vi "AWS_ConstructQuery.vi"(8 "error in (no error)":errorcluster, 11 "Queries":T1 {"Object Type" items=["File", "Channel Group", "Channel"]; "Operator" items=["=", "<>", ">", "<", ">=", "<=", "#"]}) -> (0 "error out":errorcluster, 3 "Refnum out":T4)   [LabVIEW 2014]
uses:
  <vilib>/userdefined/DFQuery.ctl
  Controls/Query.ctl
  <vilib>/DataFinder/DataTypes/object type.ctl
  <vilib>/DataFinder/DataTypes/comparison operator.ctl
  <vilib>/DataFinder/Create Query (String).vi
  <vilib>/DataFinder/Create Query (Numeric).vi
  <vilib>/DataFinder/NI_DataFinder Toolkit.lvlib
  <vilib>/userdefined/NI_DataFinder Controls.lvlib
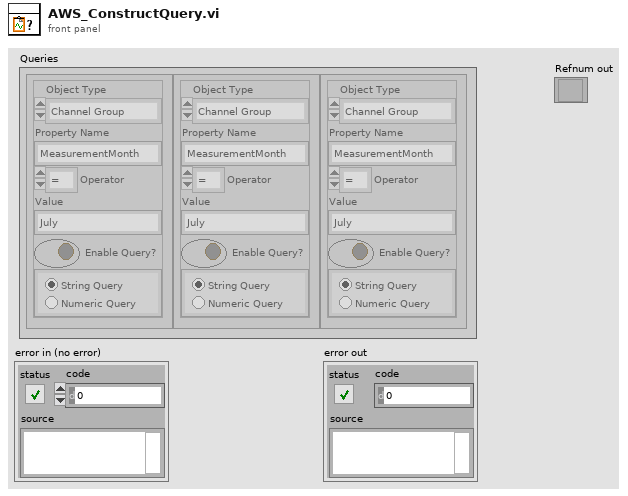
[diagram p1: front panel]
types:
  T1 = typedef "Query.ctl" = cluster{"Object Type":T2, "Property Name":string, "Operator":T3, "Value":string, "Enable Query?":bool, "Radio Buttons":enum32{"Radio Selection 1", "Radio Selection 2"}}[]
  T2 = typedef "NI_DataFinder Toolkit.lvlib/object type.ctl" = u16
  T3 = typedef "NI_DataFinder Toolkit.lvlib/comparison operator.ctl" = u16
  T4 = typedef "NI_DataFinder Controls.lvlib/DFQuery.ctl" = refnum<k20>
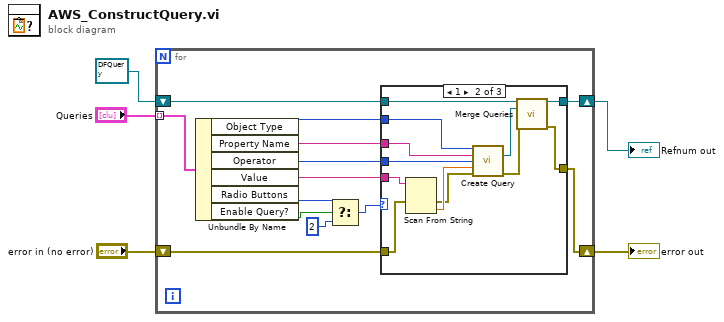
[diagram p0: block diagram]
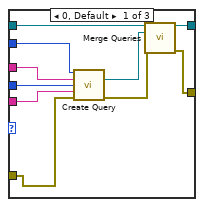
[diagram p2: hidden frame]
diagram:
  n1 = for {
    tunnel: "Queries" -> [w15] mode=indexing
    shift-right: [w17] -> w4
    shift-left: T4 refnum ("query reference out") -> [w18]
    shift-right: [w16] -> w3
    shift-left: "error in (no error)" -> [w14]
    n2 = Unbundle By Name(w15) -> ("Object Type"=w12:T2, "Property Name"=w11:string, "Operator"=w10:T3, "Value"=w13:string, "Radio Buttons"=w8:enum32{"Radio Selection 1", "Radio Selection 2"}, "Enable Query?"=w9:bool)
    n3 = Select(t=w8, s=w9, f=2) -> (s? t:f=w6:u32)
    n4 = case shown="1" w6 {
      tunnel: w13 -> [w28 w32 _]
      tunnel: w12 -> [w27 w40 _]
      tunnel: w11 -> [w26 w39 _]
      tunnel: w10 -> [w25 w38 _]
      tunnel: w18 -> [w22 w35 w42]
      tunnel: [w21 w34 w42] -> w17
      tunnel: [w20 w33 w41] -> w16
      tunnel: w14 -> [w19 w30 w41]
      frame 0, Default {
        n5 = call-poly <vilib>:"Create Query.vi"("object type"=w27, "property name"=w26, "comparison operator (=)"=w25, "value"=w28, "error in (no error)"=w19) -> ("query reference out"=w24:T4, "error out"=w23:errorcluster)  [unwired: 9 out]
        n6 = call <vilib>:"Merge Queries.vi"("query reference in 1"=w22, "query reference in 2"=w24, "error in (no error)"=w23) -> ("query reference out"=w21:T4, "error out"=w20:errorcluster)  [unwired: 2 in, 9 out]
      }
      frame 1 {
        n7 = Scan From String(input string=w32, error in=w30) -> (error out=w29:errorcluster, output 1=w31:dbl)  [unwired: 3 in, 2 out]
        n8 = call-poly <vilib>:"Create Query.vi"("object type"=w40, "property name"=w39, "comparison operator (=)"=w38, "value"=w31, "error in (no error)"=w29) -> ("query reference out"=w37:T4, "error out"=w36:errorcluster)  [unwired: 9 out]
        n9 = call <vilib>:"Merge Queries.vi"("query reference in 1"=w35, "query reference in 2"=w37, "error in (no error)"=w36) -> ("query reference out"=w34:T4, "error out"=w33:errorcluster)  [unwired: 2 in, 9 out]
      }
      frame 2 {
      }
    }
  }
  "Refnum out" <- w4
  "error out" <- w3
